vi "AddTestWithData.vi"(8 "error in (no error)":errorcluster, 10 "VI Refnum":refnum<vi>, 11 "TestSuite in":refnum<class "TestSuite.lvclass">) -> (0 "error out":errorcluster, 3 "TestSuite out":refnum<class "TestSuite.lvclass">)   [LabVIEW 2019, in "TestSuite.lvclass"]
uses:
  TestSuite.lvclass
  TestCase/Theory/Theory.lvclass
  C:/Users/de200256/Code/LVUnit/TestCase/TestCase/TestCase.lvclass
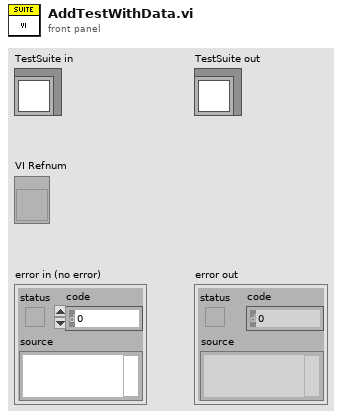
[diagram p1: front panel]
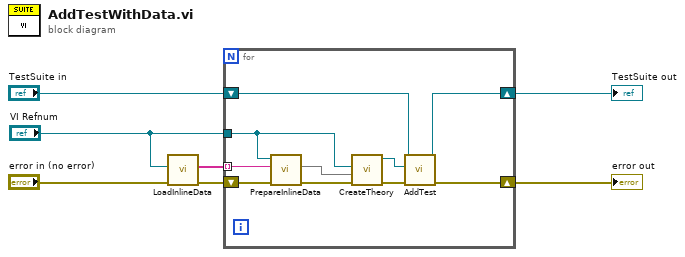
[diagram p0: block diagram]
diagram:
  n1 = call "LoadInlineData.vi"("error in (no error)"="error in (no error)", "VI Refnum"="VI Refnum") -> ("error out"=w2:errorcluster, "Inline Data"=w1:string[])  [unwired: 8 in]
  n2 = for {
    tunnel: "VI Refnum" -> [w8]
    shift-right: [w14] -> w4
    shift-left: "TestSuite in" -> [w15]
    shift-right: [w16] -> w6
    shift-left: w2 -> [w12]
    tunnel: w1 -> [w10] mode=indexing
    n3 = call "PrepareInlineData.vi"("error in (no error)"=w12, "Inline Data"=w10, "VI Refnum"=w8) -> ("error out"=w11:errorcluster, "Control Data"=w9:map{string, variant})  [unwired: 6 in, 1 out]
    n4 = call "CreateTheory.vi"("error in (no error)"=w11, "Control Data"=w9, "VI Refnum"=w8) -> ("error out"=w17:errorcluster, "Theory"=w13:refnum<class "Theory.lvclass">)  [unwired: 7 in]
    n5 = call-dynamic "AddTest.vi"("error in (no error)"=w17, "TestCase"=w13, "TestSuite in"=w15) -> ("error out"=w16:errorcluster, "TestSuite out"=w14:refnum<class "TestSuite.lvclass">)  [unwired: 7 in]
  }
  "error out" <- w6
  "TestSuite out" <- w4
